vi "ScaleFLIRAX5.vi"(7 "unit":string, 8 "error in (no error)":errorcluster, 10 "ScaledImage":T1, 11 "RawImage":T1) -> (0 "error out":errorcluster, 1 "image ok":bool, 2 "ScaledImage":T1, 4 "histogram":u32[](array[numeric]))   [LabVIEW 2017, in "IrAcquisition.lvlib"]
uses:
  <vilib>/addons/InsightCM/Devices/Shared/Ir/IrAcquisition/IrAcquisition.lvlib
  <vilib>/vision/Image Controls.llb/IMAQ Image.ctl
  <vilib>/vision/NI_Vision_Development_Module.lvlib
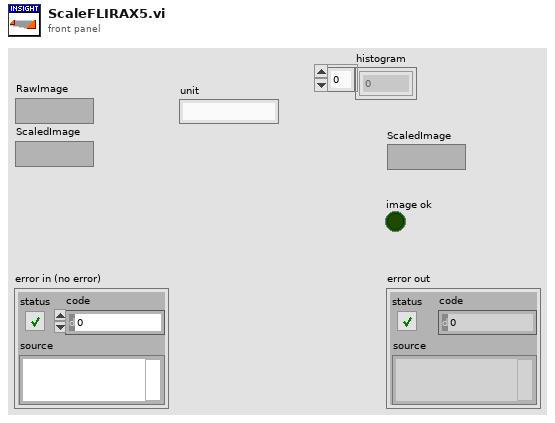
[diagram p1: front panel]
types:
  T1 = typedef "IMAQ Image.ctl" = refnum<image>
  T2 = typedef "Image Type" = u32
  T3 = cluster{"histogram":u32[], "Minimal Value":sgl, "Maximal Value":sgl, "Starting Value":sgl, "Interval Width":sgl, "Mean Value":sgl, "Standard  Variation":sgl, "Area (pixels)":i32}
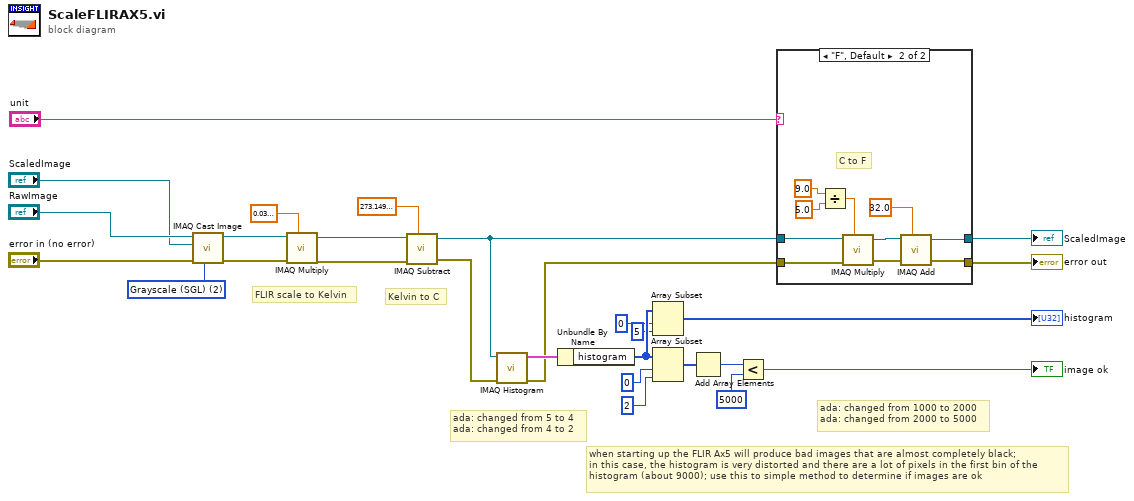
[diagram p0: block diagram]
diagram:
  w27 = T2 2 items=["Grayscale (U8)", "Grayscale (I16)", "Grayscale (SGL)", "Complex (CSG)", "RGB (U32)", "HSL (U32)", "RGB (U64)", "Grayscale (U16)"] ("Image Type")
  # "ada: changed from 1000 to 2000\nada: changed from 2000 to 5000"
  # "ada: changed from 5 to 4\nada: changed from 4 to 2"
  # "when starting up the FLIR Ax5 will produce bad images that are almost completely black;\nin this case, the histogram is very distorted and there are a lot of pixels in the first bin of the\nhistogram (about 9000); use this to simple method to determine if images are ok"
  # "Kelvin to C"
  # "FLIR scale to Kelvin"
  n1 = call "IMAQ Cast Image"("Image Type"=w27, "error in (no error)"="error in (no error)", "Image Dst"="ScaledImage", "Image Src"="RawImage") -> ("error out"=w22:errorcluster, "Image Dst Out"=w23:T1)  [unwired: 6 in]
  n2 = call "IMAQ Multiply"("Image Src A"=w23, "Constant"=sgl 0.04, "error in (no error)"=w22) -> ("Image Dst Out"=w25:T1, "error out"=w24:errorcluster)  [unwired: 4 in]
  n3 = call "IMAQ Subtract"("Image Src A"=w25, "Constant"=sgl 273.15, "error in (no error)"=w24) -> ("Image Dst Out"=w13:T1, "error out"=w12:errorcluster)  [unwired: 4 in]
  n4 = call "IMAQ Histogram"("error in (no error)"=w12, "Image"=w13) -> ("error out"=w11:errorcluster, "Histogram Report"=w14:T3)  [unwired: 8 in]
  n5 = Unbundle By Name(w14) -> ("histogram"=w4:u32[])
  n6 = Array Subset(array=w4, index=0, length=5) -> (→"histogram":u32[])
  n7 = Array Subset(array=w4, index=0, length=2 ("index")) -> (w8:u32[])
  n8 = Add Array Elements(numeric array=w8) -> (sum=w7:u32)
  n9 = Less?(x=w7, y=u32 5000) -> (x < y?=→"image ok":bool)
  n10 = case shown="\"F\", Default" "unit" {
    tunnel: [w28 w39] -> w20
    tunnel: [w29 w38] -> w15
    tunnel: w13 -> [w29 w37]
    tunnel: w11 -> [w28 w36]
    frame "C" {
    }
    frame "F", Default {
      # "C to F"
      n11 = Divide(x=9.0, y=5.0 ("x")) -> (x/y=w35:dbl)
      n12 = call "IMAQ Multiply"("Image Src A"=w37, "Constant"=w35, "error in (no error)"=w36) -> ("Image Dst Out"=w32:T1, "error out"=w31:errorcluster)  [unwired: 4 in]
      n13 = call "IMAQ Add"("Image Src A"=w32, "Constant"=sgl 32.0, "error in (no error)"=w31) -> ("Image Dst Out"=w38:T1, "error out"=w39:errorcluster)  [unwired: 4 in]
    }
  }
  "error out" <- w20
  "ScaledImage" <- w15
